vi "initialize.vi"(8 "error in (no error)":errorcluster, 11 "M1M3SAL in":refnum<class "M1M3SAL.lvclass">) -> (0 "error out":errorcluster, 3 "M1M3SAL out":refnum<class "M1M3SAL.lvclass">)   [LabVIEW 2016, in "M1M3SupportCommunicator.lvlib" / "M1M3SAL.lvclass"]
uses:
  M1M3SAL.lvclass
  M1M3SAL.lvclass/M1M3SAL.ctl
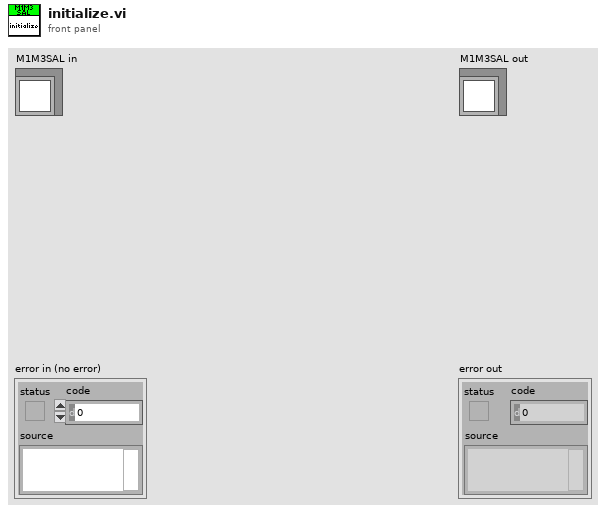
[diagram p1: front panel]
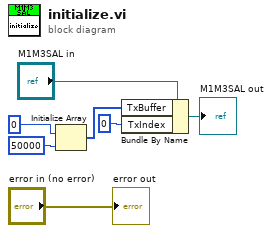
[diagram p0: block diagram]
diagram:
  n1 = Initialize Array(u8 0, 50000 ("dimension size")) -> (w4:u8[])
  n2 = Bundle By Name(cluster="M1M3SAL in", "TxBuffer"=w4, "TxIndex"=0) -> (→"M1M3SAL out":refnum<class "M1M3SAL.lvclass">)
  "error out" <- "error in (no error)"
